vi "test.vi"() -> ()   [LabVIEW 2015]
uses:
  API/JSON Document Class/json To Pretty String - string path.vi
  API/JSON Document Class/json Insert Boolean - string path.vi
  API/JSON Document Class/json Insert Path - string path.vi
  API/JSON Document Class/json Parse Path - string path.vi
  API/JSON Document Class/JSON Document.lvclass
panel:
  out "value":path
  out "json string 4":string
  out "json string 3":string
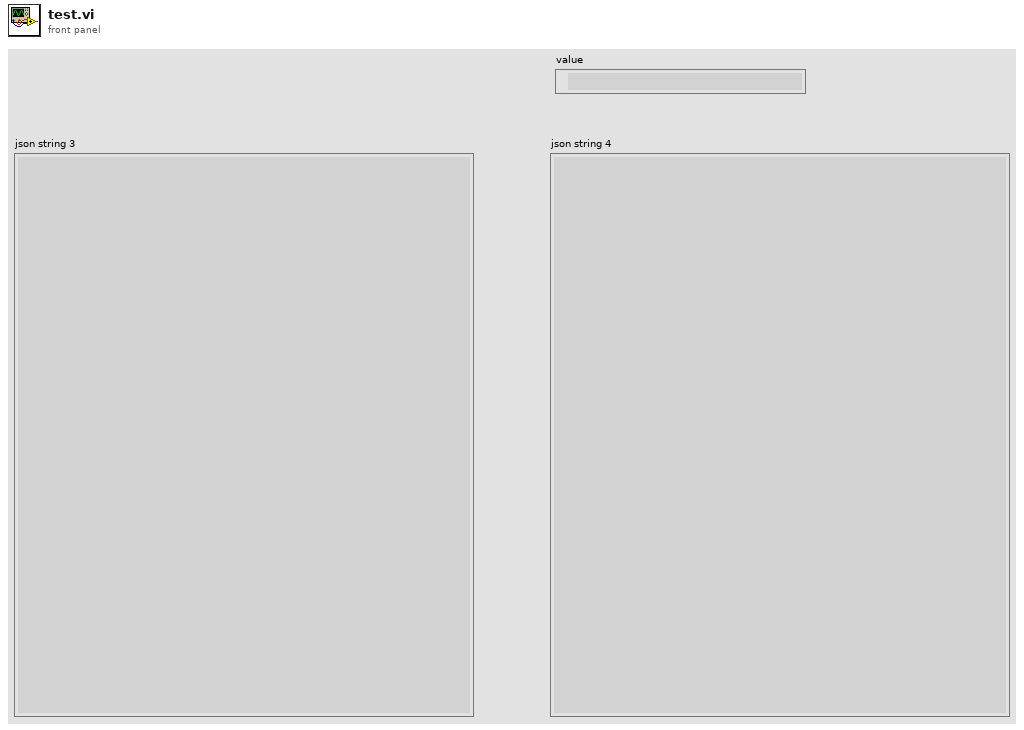
[diagram p1: front panel]
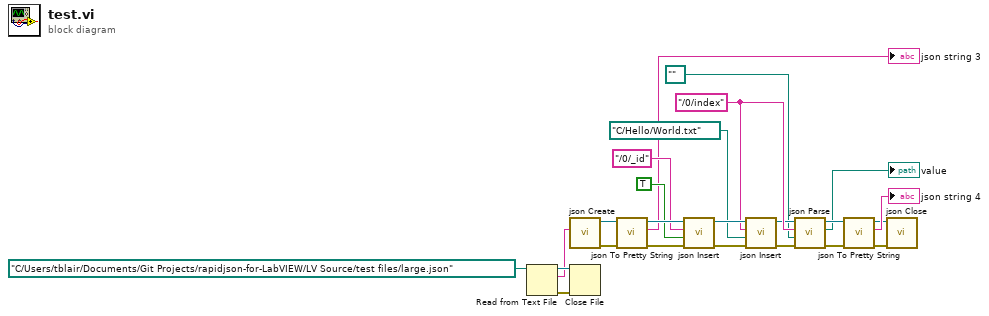
[diagram p0: block diagram]
diagram:
  w11 = "/0/index" ("path")
  n1 = Read from Text File(file (use dialog)=path "C:/Users/tblair/Documents/Git Projects/rapidjson-for-LabVIEW/LV Source/test files/large.json") -> (refnum out=w22:refnum<file>, text=w4:string, error out=w23:errorcluster)  [unwired: 3 in, 1 out]
  n2 = call "json Create.vi"("JSON String"=w4) -> ("error out"=w20:errorcluster, "JSON Document out"=w21:refnum<class "JSON Document.lvclass">)  [unwired: 9 in]
  n3 = Close File(refnum=w22, error in=w23) -> ()  [unwired: 2 out]
  n4 = call-poly "json To Pretty String.vi"("error in (no error)"=w20, "JSON Document in"=w21) -> ("error out"=w18:errorcluster, "json string"=→"json string 3":string, "JSON Document out"=w19:refnum<class "JSON Document.lvclass">)  [unwired: 7 in]
  n5 = call-poly "json Insert.vi"("error in (no error)"=w18, "anything"=TRUE, "path"="/0/_id", "JSON Document in"=w19) -> ("error out"=w15:errorcluster, "JSON Document out"=w12:refnum<class "JSON Document.lvclass">)  [unwired: 6 in]
  n6 = call-poly "json Insert.vi"("error in (no error)"=w15, "anything"=path "C:/Hello/World.txt", "path"=w11, "JSON Document in"=w12) -> ("error out"=w7:errorcluster, "JSON Document out"=w9:refnum<class "JSON Document.lvclass">)  [unwired: 6 in]
  n7 = call-poly "json Parse.vi"("error in (no error)"=w7, "default"=path "", "path"=w11, "JSON Document in"=w9) -> ("error out"=w6:errorcluster, "value"=→"value":path, "JSON Document out"=w8:refnum<class "JSON Document.lvclass">)  [unwired: 5 in]
  n8 = call-poly "json To Pretty String.vi"("error in (no error)"=w6, "JSON Document in"=w8) -> ("error out"=w5:errorcluster, "json string"=→"json string 4":string, "JSON Document out"=w10:refnum<class "JSON Document.lvclass">)  [unwired: 7 in]
  n9 = call "json Close.vi"("error in (no error)"=w5, "JSON Document in"=w10) -> ()  [unwired: 9 in, 1 out]
